vi "ConsolidatedDAQChannelNames.vi"() -> (0 "Consolidated Task Names":string, 2 "Number of \nExternal \nChannels 1":i32, 5 "LBCB2 Avalable":bool)   [LabVIEW 2013]
uses:
  Data Access Objects/Metadata/Persistant DAO Actions.ctl
  Data Access Objects/Application/Number Of LBCBs.ctl
  Data Access Objects/Metadata/LBCB Number.ctl
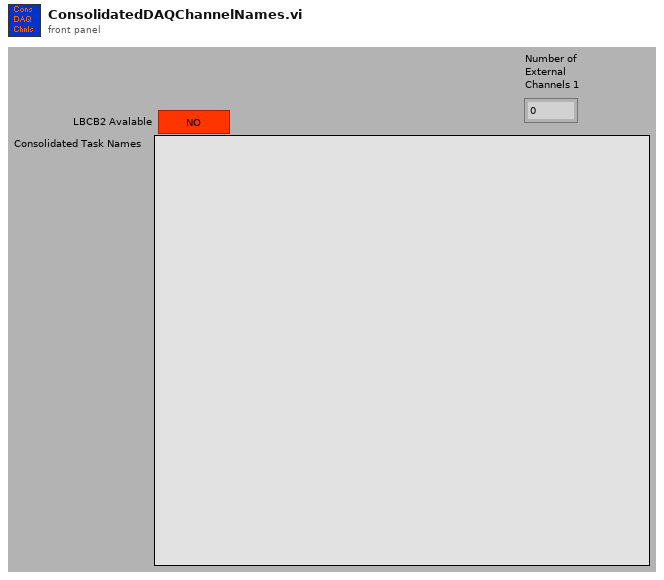
[diagram p1: front panel]
types:
  T1 = typedef "LBCB Number.ctl" = enum16{"LBCB1", "LBCB2"}
  T2 = typedef "Persistant DAO Actions.ctl" = enum16{"Init", "Get", "Set", "Load", "Save"}
  T3 = typedef "Number Of LBCBs.ctl" = enum16{"1", "2"}
  T4 = typedef "Actuator Channel Names.ctl" = cluster{"X1":refnum<k21>, "X2":refnum<k21>, "Y1":refnum<k21>, "Z1":refnum<k21>, "Z2":refnum<k21>, "Z3":refnum<k21>}
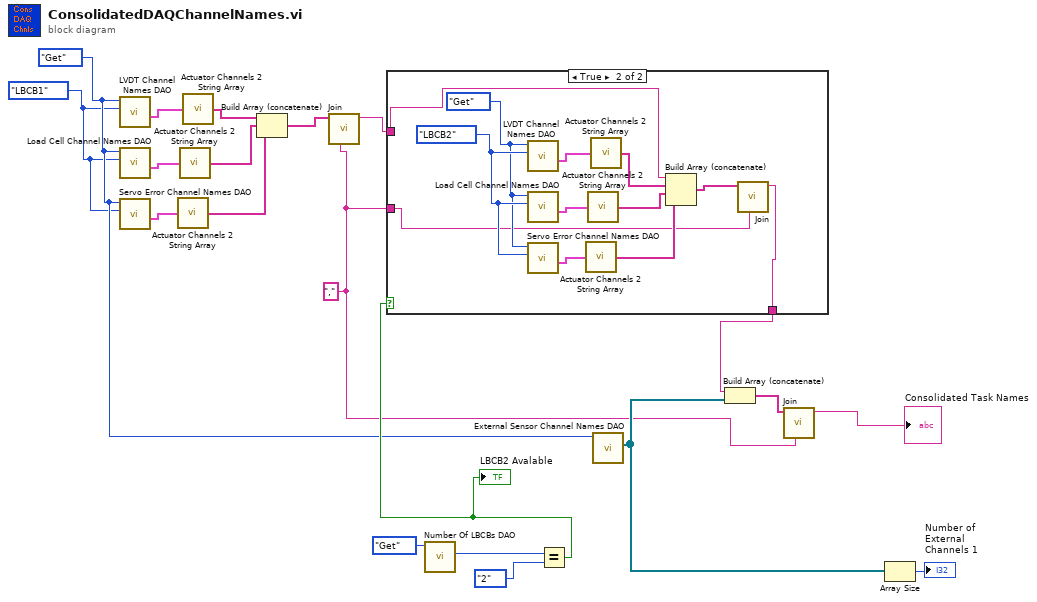
[diagram p0: block diagram]
diagram:
  w15 = LBCB_Number."LBCB1" ("LBCB Number")
  w16 = Persistant_DAO_Actions."Get" ("Actions")
  w2 = ","
  n1 = call "LVDT Channel Names DAO.vi"("LBCB Number"=w15, "Actions"=w16) -> ("Names Out"=w14:T4)  [unwired: 3 in, 6 out]
  n2 = call "Load Cell Channel Names DAO.vi"("LBCB Number"=w15, "Actions"=w16) -> ("Names Out"=w13:T4)  [unwired: 3 in, 6 out]
  n3 = call "Servo Error Channel Names DAO.vi"("LBCB Number"=w15, "Actions"=w16) -> ("Names Out"=w12:T4)  [unwired: 3 in, 6 out]
  n4 = call "Actuator Channels 2 String Array.vi"("Actuator Channels"=w12) -> ("Array"=w8:string[])
  n5 = call "Actuator Channels 2 String Array.vi"("Actuator Channels"=w13) -> ("Array"=w9:string[])
  n6 = call "Actuator Channels 2 String Array.vi"("Actuator Channels"=w14) -> ("Array"=w11:string[])
  n7 = Build Array (concatenate)(w11, w9, w8) -> (w10:string[])
  n8 = call "Join.vi"("delimiter"=w2, "Array"=w10) -> ("Joined Result"=w7:string)  [unwired: 9 out]
  n9 = call "Number Of LBCBs DAO.vi"("Actions"=Persistant_DAO_Actions."Get") -> ("Number of\nLBCBs Out"=w18:T3)  [unwired: 4 in, 6 out]
  n10 = Equal?(x=w18, y=Number_Of_LBCBs."2") -> (x = y?=w17:bool)
  "LBCB2 Avalable" <- w17
  n11 = case shown="True" w17 {
    tunnel: w2 -> [_ w24]
    tunnel: w7 -> [w21 w23]
    tunnel: [w21 w22] -> w4
    frame False {
    }
    frame True {
      w26 = LBCB_Number."LBCB2" ("LBCB Number")
      w25 = Persistant_DAO_Actions."Get" ("Actions")
      n12 = call "LVDT Channel Names DAO.vi"("LBCB Number"=w26, "Actions"=w25) -> ("Names Out"=w27:T4)  [unwired: 3 in, 6 out]
      n13 = call "Load Cell Channel Names DAO.vi"("LBCB Number"=w26, "Actions"=w25) -> ("Names Out"=w28:T4)  [unwired: 3 in, 6 out]
      n14 = call "Servo Error Channel Names DAO.vi"("LBCB Number"=w26, "Actions"=w25) -> ("Names Out"=w29:T4)  [unwired: 3 in, 6 out]
      n15 = call "Actuator Channels 2 String Array.vi"("Actuator Channels"=w29) -> ("Array"=w33:string[])
      n16 = call "Actuator Channels 2 String Array.vi"("Actuator Channels"=w28) -> ("Array"=w32:string[])
      n17 = call "Actuator Channels 2 String Array.vi"("Actuator Channels"=w27) -> ("Array"=w30:string[])
      n18 = Build Array (concatenate)(w23, w30, w32, w33) -> (w31:string[])
      n19 = call "Join.vi"("delimiter"=w24, "Array"=w31) -> ("Joined Result"=w22:string)  [unwired: 9 out]
    }
  }
  n20 = call "External Sensor Channel Names DAO.vi"("Persistent DAO Actions"=w16) -> ("DAQ Channel Out"=w3:refnum<k21>[])  [unwired: 3 in, 7 out]
  n21 = Build Array (concatenate)(w4, w3) -> (w1:string[])
  n22 = call "Join.vi"("delimiter"=w2, "Array"=w1) -> ("Joined Result"=→"Consolidated Task Names":string)  [unwired: 9 out]
  n23 = Array Size(array=w3) -> (size(s)=→"Number of \nExternal \nChannels 1":i32)
